vi "Full Complex Matrix Cholesky Factorization.vi"(0 "A":T1) -> (1 "Cholesky R":T1, 2 "error":i32)   [LabVIEW 2020, in "NI_AALBase.lvlib"]
uses:
  <vilib>/Analysis/NI_AALBase.lvlib
  <vilib>/Analysis/Matrix/Datatypes/ComplexMatrix.ctl
  <resource>/lvanlys.dll
  <vilib>/Analysis/Matrix/NI_Matrix.lvlib
panel:
  # "Full Complex Matrix Cholesky Factorization"
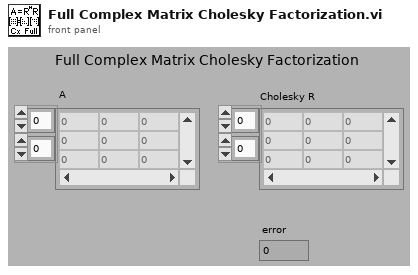
[diagram p1: front panel]
types:
  T1 = typedef "NI_Matrix.lvlib/ComplexMatrix.ctl" = cdb[][]
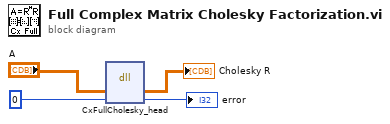
[diagram p0: block diagram]
diagram:
  n1 = dll-call lib="e:/builds/penguin/labview/branches/2020/dev/dist/resource/lvanlys.*" fn="CxFullCholesky_head"("A"="A", "error"=0) -> ("A"=→"Cholesky R":T1, "error"=→"error":i32)  [unwired: 4 in, 2 out]
